vi "App - analyze RUS V6.vi"() -> ()   [LabVIEW 2021] (continued)
s since 1904-01-01), "file name str"="D:\\Data\\Ultrasound\\LSCO\\LSCO22__130814c\\5_Cooling_2nd_try\\September_2014\\091714\\63.35500K_500_2500_2.10000V_0.00000T_Sep17-2014__07-09-10_001_091714.bin", "mod time(min)"=58229949.166666664, "file format"=enum."binary", "power(V)"=2.1, "Magn Field(T) "=0.0}, {"temperature"=63.298, "temperature str"="63.29800", "file path"=path "D:/Data/Ultrasound/LSCO/LSCO22__130814c/5_Cooling_2nd_try/September_2014/091714/63.29800K_500_2500_2.10000V_0.00000T_Sep17-2014__07-10-30_001_091714.bin", "last mod"=timestamp(3493797030 s since 1904-01-01), "file name str"="D:\\Data\\Ultrasound\\LSCO\\LSCO22__130814c\\5_Cooling_2nd_try\\September_2014\\091714\\63.29800K_500_2500_2.10000V_0.00000T_Sep17-2014__07-10-30_001_091714.bin", "mod time(min)"=58229950.5, "file format"=enum."binary", "power(V)"=2.1, "Magn Field(T) "=0.0}, {"temperature"=63.239, "temperature str"="63.23900", "file path"=path "D:/Data/Ultrasound/LSCO/LSCO22__130814c/5_Cooling_2nd_try/September_2014/091714/63.23900K_500_2500_2.10000V_0.00000T_Sep17-2014__07-11-49_001_091714.bin", "last mod"=timestamp(3493797109 s since 1904-01-01), "file name str"="D:\\Data\\Ultrasound\\LSCO\\LSCO22__130814c\\5_Cooling_2nd_try\\September_2014\\091714\\63.23900K_500_2500_2.10000V_0.00000T_Sep17-2014__07-11-49_001_091714.bin", "mod time(min)"=58229951.81666667, "file format"=enum."binary", "power(V)"=2.1, "Magn Field(T) "=0.0}, {"temperature"=63.178, "temperature str"="63.17800", "file path"=path "D:/Data/Ultrasound/LSCO/LSCO22__130814c/5_Cooling_2nd_try/September_2014/091714/63.17800K_500_2500_2.10000V_0.00000T_Sep17-2014__07-13-08_001_091714.bin", "last mod"=timestamp(3493797188 s since 1904-01-01), "file name str"="D:\\Data\\Ultrasound\\LSCO\\LSCO22__130814c\\5_Cooling_2nd_try\\September_2014\\091714\\63.17800K_500_2500_2.10000V_0.00000T_Sep17-2014__07-13-08_001_091714.bin", "mod time(min)"=58229953.13333333, "file format"=enum."binary", "power(V)"=2.1, "Magn Field(T) "=0.0}, {"temperature"=63.123, "temperature str"="63.12300", "file path"=path "D:/Data/Ultrasound/LSCO/LSCO22__130814c/5_Cooling_2nd_try/September_2014/091714/63.12300K_500_2500_2.10000V_0.00000T_Sep17-2014__07-14-28_001_091714.bin", "last mod"=timestamp(3493797268 s since 1904-01-01), "file name str"="D:\\Data\\Ultrasound\\LSCO\\LSCO22__130814c\\5_Cooling_2nd_try\\September_2014\\091714\\63.12300K_500_2500_2.10000V_0.00000T_Sep17-2014__07-14-28_001_091714.bin", "mod time(min)"=58229954.46666667, "file format"=enum."binary", "power(V)"=2.1, "Magn Field(T) "=0.0}, {"temperature"=63.063, "temperature str"="63.06300", "file path"=path "D:/Data/Ultrasound/LSCO/LSCO22__130814c/5_Cooling_2nd_try/September_2014/091714/63.06300K_500_2500_2.10000V_0.00000T_Sep17-2014__07-15-47_001_091714.bin", "last mod"=timestamp(3493797347 s since 1904-01-01), "file name str"="D:\\Data\\Ultrasound\\LSCO\\LSCO22__130814c\\5_Cooling_2nd_try\\September_2014\\091714\\63.06300K_500_2500_2.10000V_0.00000T_Sep17-2014__07-15-47_001_091714.bin", "mod time(min)"=58229955.78333333, "file format"=enum."binary", "power(V)"=2.1, "Magn Field(T) "=0.0}, {"temperature"=63.004, "temperature str"="63.00400", "file path"=path "D:/Data/Ultrasound/LSCO/LSCO22__130814c/5_Cooling_2nd_try/September_2014/091714/63.00400K_500_2500_2.10000V_0.00000T_Sep17-2014__07-17-07_001_091714.bin", "last mod"=timestamp(3493797427 s since 1904-01-01), "file name str"="D:\\Data\\Ultrasound\\LSCO\\LSCO22__130814c\\5_Cooling_2nd_try\\September_2014\\091714\\63.00400K_500_2500_2.10000V_0.00000T_Sep17-2014__07-17-07_001_091714.bin", "mod time(min)"=58229957.11666667, "file format"=enum."binary", "power(V)"=2.1, "Magn Field(T) "=0.0}, {"temperature"=62.948, "temperature str"="62.94800", "file path"=path "D:/Data/Ultrasound/LSCO/LSCO22__130814c/5_Cooling_2nd_try/September_2014/091714/62.94800K_500_2500_2.10000V_0.00000T_Sep17-2014__07-18-26_001_091714.bin", "last mod"=timestamp(3493797506 s since 1904-01-01), "file name str"="D:\\Data\\Ultrasound\\LSCO\\LSCO22__130814c\\5_Cooling_2nd_try\\September_2014\\091714\\62.94800K_500_2500_2.10000V_0.00000T_Sep17-2014__07-18-26_001_091714.bin", "mod time(min)"=58229958.43333333, "file format"=enum."binary", "power(V)"=2.1, "Magn Field(T) "=0.0}, {"temperature"=62.886, "temperature str"="62.88600", "file path"=path "D:/Data/Ultrasound/LSCO/LSCO22__130814c/5_Cooling_2nd_try/September_2014/091714/62.88600K_500_2500_2.10000V_0.00000T_Sep17-2014__07-19-45_001_091714.bin", "last mod"=timestamp(3493797585 s since 1904-01-01), "file name str"="D:\\Data\\Ultrasound\\LSCO\\LSCO22__130814c\\5_Cooling_2nd_try\\September_2014\\091714\\62.88600K_500_2500_2.10000V_0.00000T_Sep17-2014__07-19-45_001_091714.bin", "mod time(min)"=58229959.75, "file format"=enum."binary", "power(V)"=2.1, "Magn Field(T) "=0.0}, {"temperature"=62.828, "temperature str"="62.82800", "file path"=path "D:/Data/Ultrasound/LSCO/LSCO22__130814c/5_Cooling_2nd_try/September_2014/091714/62.82800K_500_2500_2.10000V_0.00000T_Sep17-2014__07-21-05_001_091714.bin", "last mod"=timestamp(3493797665 s since 1904-01-01), "file name str"="D:\\Data\\Ultrasound\\LSCO\\LSCO22__130814c\\5_Cooling_2nd_try\\September_2014\\091714\\62.82800K_500_2500_2.10000V_0.00000T_Sep17-2014__07-21-05_001_091714.bin", "mod time(min)"=58229961.083333336, "file format"=enum."binary", "power(V)"=2.1, "Magn Field(T) "=0.0}, {"temperature"=62.769, "temperature str"="62.76900", "file path"=path "D:/Data/Ultrasound/LSCO/LSCO22__130814c/5_Cooling_2nd_try/September_2014/091714/62.76900K_500_2500_2.10000V_0.00000T_Sep17-2014__07-22-24_001_091714.bin", "last mod"=timestamp(3493797744 s since 1904-01-01), "file name str"="D:\\Data\\Ultrasound\\LSCO\\LSCO22__130814c\\5_Cooling_2nd_try\\September_2014\\091714\\62.76900K_500_2500_2.10000V_0.00000T_Sep17-2014__07-22-24_001_091714.bin", "mod time(min)"=58229962.4, "file format"=enum."binary", "power(V)"=2.1, "Magn Field(T) "=0.0}, {"temperature"=62.713, "temperature str"="62.71300", "file path"=path "D:/Data/Ultrasound/LSCO/LSCO22__130814c/5_Cooling_2nd_try/September_2014/091714/62.71300K_500_2500_2.10000V_0.00000T_Sep17-2014__07-23-43_001_091714.bin", "last mod"=timestamp(3493797823 s since 1904-01-01), "file name str"="D:\\Data\\Ultrasound\\LSCO\\LSCO22__130814c\\5_Cooling_2nd_try\\September_2014\\091714\\62.71300K_500_2500_2.10000V_0.00000T_Sep17-2014__07-23-43_001_091714.bin", "mod time(min)"=58229963.71666667, "file format"=enum."binary", "power(V)"=2.1, "Magn Field(T) "=0.0}, {"temperature"=62.654, "temperature str"="62.65400", "file path"=path "D:/Data/Ultrasound/LSCO/LSCO22__130814c/5_Cooling_2nd_try/September_2014/091714/62.65400K_500_2500_2.10000V_0.00000T_Sep17-2014__07-25-03_001_091714.bin", "last mod"=timestamp(3493797903 s since 1904-01-01), "file name str"="D:\\Data\\Ultrasound\\LSCO\\LSCO22__130814c\\5_Cooling_2nd_try\\September_2014\\091714\\62.65400K_500_2500_2.10000V_0.00000T_Sep17-2014__07-25-03_001_091714.bin", "mod time(min)"=58229965.05, "file format"=enum."binary", "power(V)"=2.1, "Magn Field(T) "=0.0}, {"temperature"=62.592, "temperature str"="62.59200", "file path"=path "D:/Data/Ultrasound/LSCO/LSCO22__130814c/5_Cooling_2nd_try/September_2014/091714/62.59200K_500_2500_2.10000V_0.00000T_Sep17-2014__07-26-22_001_091714.bin", "last mod"=timestamp(3493797982 s since 1904-01-01), "file name str"="D:\\Data\\Ultrasound\\LSCO\\LSCO22__130814c\\5_Cooling_2nd_try\\September_2014\\091714\\62.59200K_500_2500_2.10000V_0.00000T_Sep17-2014__07-26-22_001_091714.bin", "mod time(min)"=58229966.36666667, "file format"=enum."binary", "power(V)"=2.1, "Magn Field(T) "=0.0}, {"temperature"=62.537, "temperature str"="62.53700", "file path"=path "D:/Data/Ultrasound/LSCO/LSCO22__130814c/5_Cooling_2nd_try/September_2014/091714/62.53700K_500_2500_2.10000V_0.00000T_Sep17-2014__07-27-42_001_091714.bin", "last mod"=timestamp(3493798062 s since 1904-01-01), "file name str"="D:\\Data\\Ultrasound\\LSCO\\LSCO22__130814c\\5_Cooling_2nd_try\\September_2014\\091714\\62.53700K_500_2500_2.10000V_0.00000T_Sep17-2014__07-27-42_001_091714.bin", "mod time(min)"=58229967.7, "file format"=enum."binary", "power(V)"=2.1, "Magn Field(T) "=0.0}, {"temperature"=62.48, "temperature str"="62.48000", "file path"=path "D:/Data/Ultrasound/LSCO/LSCO22__130814c/5_Cooling_2nd_try/September_2014/091714/62.48000K_500_2500_2.10000V_0.00000T_Sep17-2014__07-29-01_001_091714.bin", "last mod"=timestamp(3493798141 s since 1904-01-01), "file name str"="D:\\Data\\Ultrasound\\LSCO\\LSCO22__130814c\\5_Cooling_2nd_try\\September_2014\\091714\\62.48000K_500_2500_2.10000V_0.00000T_Sep17-2014__07-29-01_001_091714.bin", "mod time(min)"=58229969.016666666, "file format"=enum."binary", "power(V)"=2.1, "Magn Field(T) "=0.0}, {"temperature"=62.42, "temperature str"="62.42000", "file path"=path "D:/Data/Ultrasound/LSCO/LSCO22__130814c/5_Cooling_2nd_try/September_2014/091714/62.42000K_500_2500_2.10000V_0.00000T_Sep17-2014__07-30-20_001_091714.bin", "last mod"=timestamp(3493798220 s since 1904-01-01), "file name str"="D:\\Data\\Ultrasound\\LSCO\\LSCO22__130814c\\5_Cooling_2nd_try\\September_2014\\091714\\62.42000K_500_2500_2.10000V_0.00000T_Sep17-2014__07-30-20_001_091714.bin", "mod time(min)"=58229970.333333336, "file format"=enum."binary", "power(V)"=2.1, "Magn Field(T) "=0.0}, {"temperature"=62.361, "temperature str"="62.36100", "file path"=path "D:/Data/Ultrasound/LSCO/LSCO22__130814c/5_Cooling_2nd_try/September_2014/091714/62.36100K_500_2500_2.10000V_0.00000T_Sep17-2014__07-31-40_001_091714.bin", "last mod"=timestamp(3493798300 s since 1904-01-01), "file name str"="D:\\Data\\Ultrasound\\LSCO\\LSCO22__130814c\\5_Cooling_2nd_try\\September_2014\\091714\\62.36100K_500_2500_2.10000V_0.00000T_Sep17-2014__07-31-40_001_091714.bin", "mod time(min)"=58229971.666666664, "file format"=enum."binary", "power(V)"=2.1, "Magn Field(T) "=0.0}, {"temperature"=62.301, "temperature str"="62.30100", "file path"=path "D:/Data/Ultrasound/LSCO/LSCO22__130814c/5_Cooling_2nd_try/September_2014/091714/62.30100K_500_2500_2.10000V_0.00000T_Sep17-2014__07-32-59_001_091714.bin", "last mod"=timestamp(3493798379 s since 1904-01-01), "file name str"="D:\\Data\\Ultrasound\\LSCO\\LSCO22__130814c\\5_Cooling_2nd_try\\September_2014\\091714\\62.30100K_500_2500_2.10000V_0.00000T_Sep17-2014__07-32-59_001_091714.bin", "mod time(min)"=58229972.983333334, "file format"=enum."binary", "power(V)"=2.1, "Magn Field(T) "=0.0}, {"temperature"=62.245, "temperature str"="62.24500", "file path"=path "D:/Data/Ultrasound/LSCO/LSCO22__130814c/5_Cooling_2nd_try/September_2014/091714/62.24500K_500_2500_2.10000V_0.00000T_Sep17-2014__07-34-19_001_091714.bin", "last mod"=timestamp(3493798459 s since 1904-01-01), "file name str"="D:\\Data\\Ultrasound\\LSCO\\LSCO22__130814c\\5_Cooling_2nd_try\\September_2014\\091714\\62.24500K_500_2500_2.10000V_0.00000T_Sep17-2014__07-34-19_001_091714.bin", "mod time(min)"=58229974.31666667, "file format"=enum."binary", "power(V)"=2.1, "Magn Field(T) "=0.0}, {"temperature"=62.184, "temperature str"="62.18400", "file path"=path "D:/Data/Ultrasound/LSCO/LSCO22__130814c/5_Cooling_2nd_try/September_2014/091714/62.18400K_500_2500_2.10000V_0.00000T_Sep17-2014__07-35-38_001_091714.bin", "last mod"=timestamp(3493798538 s since 1904-01-01), "file name str"="D:\\Data\\Ultrasound\\LSCO\\LSCO22__130814c\\5_Cooling_2nd_try\\September_2014\\091714\\62.18400K_500_2500_2.10000V_0.00000T_Sep17-2014__07-35-38_001_091714.bin", "mod time(min)"=58229975.63333333, "file format"=enum."binary", "power(V)"=2.1, "Magn Field(T) "=0.0}, {"temperature"=62.127, "temperature str"="62.12700", "file path"=path "D:/Data/Ultrasound/LSCO/LSCO22__130814c/5_Cooling_2nd_try/September_2014/091714/62.12700K_500_2500_2.10000V_0.00000T_Sep17-2014__07-36-57_001_091714.bin", "last mod"=timestamp(3493798617 s since 1904-01-01), "file name str"="D:\\Data\\Ultrasound\\LSCO\\LSCO22__130814c\\5_Cooling_2nd_try\\September_2014\\091714\\62.12700K_500_2500_2.10000V_0.00000T_Sep17-2014__07-36-57_001_091714.bin", "mod time(min)"=58229976.95, "file format"=enum."binary", "power(V)"=2.1, "Magn Field(T) "=0.0}, {"temperature"=62.069, "temperature str"="62.06900", "file path"=path "D:/Data/Ultrasound/LSCO/LSCO22__130814c/5_Cooling_2nd_try/September_2014/091714/62.06900K_500_2500_2.10000V_0.00000T_Sep17-2014__07-38-17_001_091714.bin", "last mod"=timestamp(3493798697 s since 1904-01-01), "file name str"="D:\\Data\\Ultrasound\\LSCO\\LSCO22__130814c\\5_Cooling_2nd_try\\September_2014\\091714\\62.06900K_500_2500_2.10000V_0.00000T_Sep17-2014__07-38-17_001_091714.bin", "mod time(min)"=58229978.28333333, "file format"=enum."binary", "power(V)"=2.1, "Magn Field(T) "=0.0}, {"temperature"=62.01, "temperature str"="62.01000", "file path"=path "D:/Data/Ultrasound/LSCO/LSCO22__130814c/5_Cooling_2nd_try/September_2014/091714/62.01000K_500_2500_2.10000V_0.00000T_Sep17-2014__07-39-36_001_091714.bin", "last mod"=timestamp(3493798776 s since 1904-01-01), "file name str"="D:\\Data\\Ultrasound\\LSCO\\LSCO22__130814c\\5_Cooling_2nd_try\\September_2014\\091714\\62.01000K_500_2500_2.10000V_0.00000T_Sep17-2014__07-39-36_001_091714.bin", "mod time(min)"=58229979.6, "file format"=enum."binary", "power(V)"=2.1, "Magn Field(T) "=0.0}, {"temperature"=61.951, "temperature str"="61.95100", "file path"=path "D:/Data/Ultrasound/LSCO/LSCO22__130814c/5_Cooling_2nd_try/September_2014/091714/61.95100K_500_2500_2.10000V_0.00000T_Sep17-2014__07-40-55_001_091714.bin", "last mod"=timestamp(3493798855 s since 1904-01-01), "file name str"="D:\\Data\\Ultrasound\\LSCO\\LSCO22__130814c\\5_Cooling_2nd_try\\September_2014\\091714\\61.95100K_500_2500_2.10000V_0.00000T_Sep17-2014__07-40-55_001_091714.bin", "mod time(min)"=58229980.916666664, "file format"=enum."binary", "power(V)"=2.1, "Magn Field(T) "=0.0}, {"temperature"=61.895, "temperature str"="61.89500", "file path"=path "D:/Data/Ultrasound/LSCO/LSCO22__130814c/5_Cooling_2nd_try/September_2014/091714/61.89500K_500_2500_2.10000V_0.00000T_Sep17-2014__07-42-15_001_091714.bin", "last mod"=timestamp(3493798935 s since 1904-01-01), "file name str"="D:\\Data\\Ultrasound\\LSCO\\LSCO22__130814c\\5_Cooling_2nd_try\\September_2014\\091714\\61.89500K_500_2500_2.10000V_0.00000T_Sep17-2014__07-42-15_001_091714.bin", "mod time(min)"=58229982.25, "file format"=enum."binary", "power(V)"=2.1, "Magn Field(T) "=0.0}, {"temperature"=61.834, "temperature str"="61.83400", "file path"=path "D:/Data/Ultrasound/LSCO/LSCO22__130814c/5_Cooling_2nd_try/September_2014/091714/61.83400K_500_2500_2.10000V_0.00000T_Sep17-2014__07-43-34_001_091714.bin", "last mod"=timestamp(3493799014 s since 1904-01-01), "file name str"="D:\\Data\\Ultrasound\\LSCO\\LSCO22__130814c\\5_Cooling_2nd_try\\September_2014\\091714\\61.83400K_500_2500_2.10000V_0.00000T_Sep17-2014__07-43-34_001_091714.bin", "mod time(min)"=58229983.56666667, "file format"=enum."binary", "power(V)"=2.1, "Magn Field(T) "=0.0}, {"temperature"=61.775, "temperature str"="61.77500", "file path"=path "D:/Data/Ultrasound/LSCO/LSCO22__130814c/5_Cooling_2nd_try/September_2014/091714/61.77500K_500_2500_2.10000V_0.00000T_Sep17-2014__07-44-54_001_091714.bin", "last mod"=timestamp(3493799094 s since 1904-01-01), "file name str"="D:\\Data\\Ultrasound\\LSCO\\LSCO22__130814c\\5_Cooling_2nd_try\\September_2014\\091714\\61.77500K_500_2500_2.10000V_0.00000T_Sep17-2014__07-44-54_001_091714.bin", "mod time(min)"=58229984.9, "file format"=enum."binary", "power(V)"=2.1, "Magn Field(T) "=0.0}, {"temperature"=61.716, "temperature str"="61.71600", "file path"=path "D:/Data/Ultrasound/LSCO/LSCO22__130814c/5_Cooling_2nd_try/September_2014/091714/61.71600K_500_2500_2.10000V_0.00000T_Sep17-2014__07-46-13_001_091714.bin", "last mod"=timestamp(3493799173 s since 1904-01-01), "file name str"="D:\\Data\\Ultrasound\\LSCO\\LSCO22__130814c\\5_Cooling_2nd_try\\September_2014\\091714\\61.71600K_500_2500_2.10000V_0.00000T_Sep17-2014__07-46-13_001_091714.bin", "mod time(min)"=58229986.21666667, "file format"=enum."binary", "power(V)"=2.1, "Magn Field(T) "=0.0}, {"temperature"=61.656, "temperature str"="61.65600", "file path"=path "D:/Data/Ultrasound/LSCO/LSCO22__130814c/5_Cooling_2nd_try/September_2014/091714/61.65600K_500_2500_2.10000V_0.00000T_Sep17-2014__07-47-32_001_091714.bin", "last mod"=timestamp(3493799252 s since 1904-01-01), "file name str"="D:\\Data\\Ultrasound\\LSCO\\LSCO22__130814c\\5_Cooling_2nd_try\\September_2014\\091714\\61.65600K_500_2500_2.10000V_0.00000T_Sep17-2014__07-47-32_001_091714.bin", "mod time(min)"=58229987.53333333, "file format"=enum."binary", "power(V)"=2.1, "Magn Field(T) "=0.0}, {"temperature"=61.601, "temperature str"="61.60100", "file path"=path "D:/Data/Ultrasound/LSCO/LSCO22__130814c/5_Cooling_2nd_try/September_2014/091714/61.60100K_500_2500_2.10000V_0.00000T_Sep17-2014__07-48-52_001_091714.bin", "last mod"=timestamp(3493799332 s since 1904-01-01), "file name str"="D:\\Data\\Ultrasound\\LSCO\\LSCO22__130814c\\5_Cooling_2nd_try\\September_2014\\091714\\61.60100K_500_2500_2.10000V_0.00000T_Sep17-2014__07-48-52_001_091714.bin", "mod time(min)"=58229988.86666667, "file format"=enum."binary", "power(V)"=2.1, "Magn Field(T) "=0.0}, {"temperature"=61.541, "temperature str"="61.54100", "file path"=path "D:/Data/Ultrasound/LSCO/LSCO22__130814c/5_Cooling_2nd_try/September_2014/091714/61.54100K_500_2500_2.10000V_0.00000T_Sep17-2014__07-50-11_001_091714.bin", "last mod"=timestamp(3493799411 s since 1904-01-01), "file name str"="D:\\Data\\Ultrasound\\LSCO\\LSCO22__130814c\\5_Cooling_2nd_try\\September_2014\\091714\\61.54100K_500_2500_2.10000V_0.00000T_Sep17-2014__07-50-11_001_091714.bin", "mod time(min)"=58229990.18333333, "file format"=enum."binary", "power(V)"=2.1, "Magn Field(T) "=0.0}, {"temperature"=61.482, "temperature str"="61.48200", "file path"=path "D:/Data/Ultrasound/LSCO/LSCO22__130814c/5_Cooling_2nd_try/September_2014/091714/61.48200K_500_2500_2.10000V_0.00000T_Sep17-2014__07-51-31_001_091714.bin", "last mod"=timestamp(3493799491 s since 1904-01-01), "file name str"="D:\\Data\\Ultrasound\\LSCO\\LSCO22__130814c\\5_Cooling_2nd_try\\September_2014\\091714\\61.48200K_500_2500_2.10000V_0.00000T_Sep17-2014__07-51-31_001_091714.bin", "mod time(min)"=58229991.516666666, "file format"=enum."binary", "power(V)"=2.1, "Magn Field(T) "=0.0}, {"temperature"=61.424, "temperature str"="61.42400", "file path"=path "D:/Data/Ultrasound/LSCO/LSCO22__130814c/5_Cooling_2nd_try/September_2014/091714/61.42400K_500_2500_2.10000V_0.00000T_Sep17-2014__07-52-50_001_091714.bin", "last mod"=timestamp(3493799570 s since 1904-01-01), "file name str"="D:\\Data\\Ultrasound\\LSCO\\LSCO22__130814c\\5_Cooling_2nd_try\\September_2014\\091714\\61.42400K_500_2500_2.10000V_0.00000T_Sep17-2014__07-52-50_001_091714.bin", "mod time(min)"=58229992.833333336, "file format"=enum."binary", "power(V)"=2.1, "Magn Field(T) "=0.0}, {"temperature"=61.367, "temperature str"="61.36700", "file path"=path "D:/Data/Ultrasound/LSCO/LSCO22__130814c/5_Cooling_2nd_try/September_2014/091714/61.36700K_500_2500_2.10000V_0.00000T_Sep17-2014__07-54-09_001_091714.bin", "last mod"=timestamp(3493799649 s since 1904-01-01), "file name str"="D:\\Data\\Ultrasound\\LSCO\\LSCO22__130814c\\5_Cooling_2nd_try\\September_2014\\091714\\61.36700K_500_2500_2.10000V_0.00000T_Sep17-2014__07-54-09_001_091714.bin", "mod time(min)"=58229994.15, "file format"=enum."binary", "power(V)"=2.1, "Magn Field(T) "=0.0}, {"temperature"=61.307, "temperature str"="61.30700", "file path"=path "D:/Data/Ultrasound/LSCO/LSCO22__130814c/5_Cooling_2nd_try/September_2014/091714/61.30700K_500_2500_2.10000V_0.00000T_Sep17-2014__07-55-29_001_091714.bin", "last mod"=timestamp(3493799729 s since 1904-01-01), "file name str"="D:\\Data\\Ultrasound\\LSCO\\LSCO22__130814c\\5_Cooling_2nd_try\\September_2014\\091714\\61.30700K_500_2500_2.10000V_0.00000T_Sep17-2014__07-55-29_001_091714.bin", "mod time(min)"=58229995.483333334, "file format"=enum."binary", "power(V)"=2.1, "Magn Field(T) "=0.0}, {"temperature"=61.247, "temperature str"="61.24700", "file path"=path "D:/Data/Ultrasound/LSCO/LSCO22__130814c/5_Cooling_2nd_try/September_2014/091714/61.24700K_500_2500_2.10000V_0.00000T_Sep17-2014__07-56-48_001_091714.bin", "last mod"=timestamp(3493799808 s since 1904-01-01), "file name str"="D:\\Data\\Ultrasound\\LSCO\\LSCO22__130814c\\5_Cooling_2nd_try\\September_2014\\091714\\61.24700K_500_2500_2.10000V_0.00000T_Sep17-2014__07-56-48_001_091714.bin", "mod time(min)"=58229996.8, "file format"=enum."binary", "power(V)"=2.1, "Magn Field(T) "=0.0}, {"temperature"=61.191, "temperature str"="61.19100", "file path"=path "D:/Data/Ultrasound/LSCO/LSCO22__130814c/5_Cooling_2nd_try/September_2014/091714/61.19100K_500_2500_2.10000V_0.00000T_Sep17-2014__07-58-07_001_091714.bin", "last mod"=timestamp(3493799887 s since 1904-01-01), "file name str"="D:\\Data\\Ultrasound\\LSCO\\LSCO22__130814c\\5_Cooling_2nd_try\\September_2014\\091714\\61.19100K_500_2500_2.10000V_0.00000T_Sep17-2014__07-58-07_001_091714.bin", "mod time(min)"=58229998.11666667, "file format"=enum."binary", "power(V)"=2.1, "Magn Field(T) "=0.0}, {"temperature"=61.13, "temperature str"="61.13000", "file path"=path "D:/Data/Ultrasound/LSCO/LSCO22__130814c/5_Cooling_2nd_try/September_2014/091714/61.13000K_500_2500_2.10000V_0.00000T_Sep17-2014__07-59-27_001_091714.bin", "last mod"=timestamp(3493799967 s since 1904-01-01), "file name str"="D:\\Data\\Ultrasound\\LSCO\\LSCO22__130814c\\5_Cooling_2nd_try\\September_2014\\091714\\61.13000K_500_2500_2.10000V_0.00000T_Sep17-2014__07-59-27_001_091714.bin", "mod time(min)"=58229999.45, "file format"=enum."binary", "power(V)"=2.1, "Magn Field(T) "=0.0}, {"temperature"=61.073, "temperature str"="61.07300", "file path"=path "D:/Data/Ultrasound/LSCO/LSCO22__130814c/5_Cooling_2nd_try/September_2014/091714/61.07300K_500_2500_2.10000V_0.00000T_Sep17-2014__08-00-46_001_091714.bin", "last mod"=timestamp(3493800046 s since 1904-01-01), "file name str"="D:\\Data\\Ultrasound\\LSCO\\LSCO22__130814c\\5_Cooling_2nd_try\\September_2014\\091714\\61.07300K_500_2500_2.10000V_0.00000T_Sep17-2014__08-00-46_001_091714.bin", "mod time(min)"=58230000.766666666, "file format"=enum."binary", "power(V)"=2.1, "Magn Field(T) "=0.0}, {"temperature"=61.013, "temperature str"="61.01300", "file path"=path "D:/Data/Ultrasound/LSCO/LSCO22__130814c/5_Cooling_2nd_try/September_2014/091714/61.01300K_500_2500_2.10000V_0.00000T_Sep17-2014__08-02-06_001_091714.bin", "last mod"=timestamp(3493800126 s since 1904-01-01), "file name str"="D:\\Data\\Ultrasound\\LSCO\\LSCO22__130814c\\5_Cooling_2nd_try\\September_2014\\091714\\61.01300K_500_2500_2.10000V_0.00000T_Sep17-2014__08-02-06_001_091714.bin", "mod time(min)"=58230002.1, "file format"=enum."binary", "power(V)"=2.1, "Magn Field(T) "=0.0}, {"temperature"=60.953, "temperature str"="60.95300", "file path"=path "D:/Data/Ultrasound/LSCO/LSCO22__130814c/5_Cooling_2nd_try/September_2014/091714/60.95300K_500_2500_2.10000V_0.00000T_Sep17-2014__08-03-25_001_091714.bin", "last mod"=timestamp(3493800205 s since 1904-01-01), "file name str"="D:\\Data\\Ultrasound\\LSCO\\LSCO22__130814c\\5_Cooling_2nd_try\\September_2014\\091714\\60.95300K_500_2500_2.10000V_0.00000T_Sep17-2014__08-03-25_001_091714.bin", "mod time(min)"=58230003.416666664, "file format"=enum."binary", "power(V)"=2.1, "Magn Field(T) "=0.0}, {"temperature"=60.896, "temperature str"="60.89600", "file path"=path "D:/Data/Ultrasound/LSCO/LSCO22__130814c/5_Cooling_2nd_try/September_2014/091714/60.89600K_500_2500_2.10000V_0.00000T_Sep17-2014__08-04-44_001_091714.bin", "last mod"=timestamp(3493800284 s since 1904-01-01), "file name str"="D:\\Data\\Ultrasound\\LSCO\\LSCO22__130814c\\5_Cooling_2nd_try\\September_2014\\091714\\60.89600K_500_2500_2.10000V_0.00000T_Sep17-2014__08-04-44_001_091714.bin", "mod time(min)"=58230004.733333334, "file format"=enum."binary", "power(V)"=2.1, "Magn Field(T) "=0.0}, {"temperature"=60.837, "temperature str"="60.83700", "file path"=path "D:/Data/Ultrasound/LSCO/LSCO22__130814c/5_Cooling_2nd_try/September_2014/091714/60.83700K_500_2500_2.10000V_0.00000T_Sep17-2014__08-06-04_001_091714.bin", "last mod"=timestamp(3493800364 s since 1904-01-01), "file name str"="D:\\Data\\Ultrasound\\LSCO\\LSCO22__130814c\\5_Cooling_2nd_try\\September_2014\\091714\\60.83700K_500_2500_2.10000V_0.00000T_Sep17-2014__08-06-04_001_091714.bin", "mod time(min)"=58230006.06666667, "file format"=enum."binary", "power(V)"=2.1, "Magn Field(T) "=0.0}, {"temperature"=60.781, "temperature str"="60.78100", "file path"=path "D:/Data/Ultrasound/LSCO/LSCO22__130814c/5_Cooling_2nd_try/September_2014/091714/60.78100K_500_2500_2.10000V_0.00000T_Sep17-2014__08-07-23_001_091714.bin", "last mod"=timestamp(3493800443 s since 1904-01-01), "file name str"="D:\\Data\\Ultrasound\\LSCO\\LSCO22__130814c\\5_Cooling_2nd_try\\September_2014\\091714\\60.78100K_500_2500_2.10000V_0.00000T_Sep17-2014__08-07-23_001_091714.bin", "mod time(min)"=58230007.38333333, "file format"=enum."binary", "power(V)"=2.1, "Magn Field(T) "=0.0}, {"temperature"=60.72, "temperature str"="60.72000", "file path"=path "D:/Data/Ultrasound/LSCO/LSCO22__130814c/5_Cooling_2nd_try/September_2014/091714/60.72000K_500_2500_2.10000V_0.00000T_Sep17-2014__08-08-42_001_091714.bin", "last mod"=timestamp(3493800522 s since 1904-01-01), "file name str"="D:\\Data\\Ultrasound\\LSCO\\LSCO22__130814c\\5_Cooling_2nd_try\\September_2014\\091714\\60.72000K_500_2500_2.10000V_0.00000T_Sep17-2014__08-08-42_001_091714.bin", "mod time(min)"=58230008.7, "file format"=enum."binary", "power(V)"=2.1, "Magn Field(T) "=0.0}, {"temperature"=60.659, "temperature str"="60.65900", "file path"=path "D:/Data/Ultrasound/LSCO/LSCO22__130814c/5_Cooling_2nd_try/September_2014/091714/60.65900K_500_2500_2.10000V_0.00000T_Sep17-2014__08-10-02_001_091714.bin", "last mod"=timestamp(3493800602 s since 1904-01-01), "file name str"="D:\\Data\\Ultrasound\\LSCO\\LSCO22__130814c\\5_Cooling_2nd_try\\September_2014\\091714\\60.65900K_500_2500_2.10000V_0.00000T_Sep17-2014__08-10-02_001_091714.bin", "mod time(min)"=58230010.03333333, "file format"=enum."binary", "power(V)"=2.1, "Magn Field(T) "=0.0}, {"temperature"=60.601, "temperature str"="60.60100", "file path"=path "D:/Data/Ultrasound/LSCO/LSCO22__130814c/5_Cooling_2nd_try/September_2014/091714/60.60100K_500_2500_2.10000V_0.00000T_Sep17-2014__08-11-21_001_091714.bin", "last mod"=timestamp(3493800681 s since 1904-01-01), "file name str"="D:\\Data\\Ultrasound\\LSCO\\LSCO22__130814c\\5_Cooling_2nd_try\\September_2014\\091714\\60.60100K_500_2500_2.10000V_0.00000T_Sep17-2014__08-11-21_001_091714.bin", "mod time(min)"=58230011.35, "file format"=enum."binary", "power(V)"=2.1, "Magn Field(T) "=0.0}, {"temperature"=60.545, "temperature str"="60.54500", "file path"=path "D:/Data/Ultrasound/LSCO/LSCO22__130814c/5_Cooling_2nd_try/September_2014/091714/60.54500K_500_2500_2.10000V_0.00000T_Sep17-2014__08-12-41_001_091714.bin", "last mod"=timestamp(3493800761 s since 1904-01-01), "file name str"="D:\\Data\\Ultrasound\\LSCO\\LSCO22__130814c\\5_Cooling_2nd_try\\September_2014\\091714\\60.54500K_500_2500_2.10000V_0.00000T_Sep17-2014__08-12-41_001_091714.bin", "mod time(min)"=58230012.68333333, "file format"=enum."binary", "power(V)"=2.1, "Magn Field(T) "=0.0}, {"temperature"=60.486, "temperature str"="60.48600", "file path"=path "D:/Data/Ultrasound/LSCO/LSCO22__130814c/5_Cooling_2nd_try/September_2014/091714/60.48600K_500_2500_2.10000V_0.00000T_Sep17-2014__08-14-00_001_091714.bin", "last mod"=timestamp(3493800840 s since 1904-01-01), "file name str"="D:\\Data\\Ultrasound\\LSCO\\LSCO22__130814c\\5_Cooling_2nd_try\\September_2014\\091714\\60.48600K_500_2500_2.10000V_0.00000T_Sep17-2014__08-14-00_001_091714.bin", "mod time(min)"=58230014.0, "file format"=enum."binary", "power(V)"=2.1, "Magn Field(T) "=0.0}, {"temperature"=60.426, "temperature str"="60.42600", "file path"=path "D:/Data/Ultrasound/LSCO/LSCO22__130814c/5_Cooling_2nd_try/September_2014/091714/60.42600K_500_2500_2.10000V_0.00000T_Sep17-2014__08-15-19_001_091714.bin", "last mod"=timestamp(3493800919 s since 1904-01-01), "file name str"="D:\\Data\\Ultrasound\\LSCO\\LSCO22__130814c\\5_Cooling_2nd_try\\September_2014\\091714\\60.42600K_500_2500_2.10000V_0.00000T_Sep17-2014__08-15-19_001_091714.bin", "mod time(min)"=58230015.31666667, "file format"=enum."binary", "power(V)"=2.1, "Magn Field(T) "=0.0}, {"temperature"=60.367, "temperature str"="60.36700", "file path"=path "D:/Data/Ultrasound/LSCO/LSCO22__130814c/5_Cooling_2nd_try/September_2014/091714/60.36700K_500_2500_2.10000V_0.00000T_Sep17-2014__08-16-39_001_091714.bin", "last mod"=timestamp(3493800999 s since 1904-01-01), "file name str"="D:\\Data\\Ultrasound\\LSCO\\LSCO22__130814c\\5_Cooling_2nd_try\\September_2014\\091714\\60.36700K_500_2500_2.10000V_0.00000T_Sep17-2014__08-16-39_001_091714.bin", "mod time(min)"=58230016.65, "file format"=enum."binary", "power(V)"=2.1, "Magn Field(T) "=0.0}, {"temperature"=60.308, "temperature str"="60.30800", "file path"=path "D:/Data/Ultrasound/LSCO/LSCO22__130814c/5_Cooling_2nd_try/September_2014/091714/60.30800K_500_2500_2.10000V_0.00000T_Sep17-2014__08-17-58_001_091714.bin", "last mod"=timestamp(3493801078 s since 1904-01-01), "file name str"="D:\\Data\\Ultrasound\\LSCO\\LSCO22__130814c\\5_Cooling_2nd_try\\September_2014\\091714\\60.30800K_500_2500_2.10000V_0.00000T_Sep17-2014__08-17-58_001_091714.bin", "mod time(min)"=58230017.96666667, "file format"=enum."binary", "power(V)"=2.1, "Magn Field(T) "=0.0}, {"temperature"=60.248, "temperature str"="60.24800", "file path"=path "D:/Data/Ultrasound/LSCO/LSCO22__130814c/5_Cooling_2nd_try/September_2014/091714/60.24800K_500_2500_2.10000V_0.00000T_Sep17-2014__08-19-18_001_091714.bin", "last mod"=timestamp(3493801158 s since 1904-01-01), "file name str"="D:\\Data\\Ultrasound\\LSCO\\LSCO22__130814c\\5_Cooling_2nd_try\\September_2014\\091714\\60.24800K_500_2500_2.10000V_0.00000T_Sep17-2014__08-19-18_001_091714.bin", "mod time(min)"=58230019.3, "file format"=enum."binary", "power(V)"=2.1, "Magn Field(T) "=0.0}, {"temperature"=60.19, "temperature str"="60.19000", "file path"=path "D:/Data/Ultrasound/LSCO/LSCO22__130814c/5_Cooling_2nd_try/September_2014/091714/60.19000K_500_2500_2.10000V_0.00000T_Sep17-2014__08-20-37_001_091714.bin", "last mod"=timestamp(3493801237 s since 1904-01-01), "file name str"="D:\\Data\\Ultrasound\\LSCO\\LSCO22__130814c\\5_Cooling_2nd_try\\September_2014\\091714\\60.19000K_500_2500_2.10000V_0.00000T_Sep17-2014__08-20-37_001_091714.bin", "mod time(min)"=58230020.61666667, "file format"=enum."binary", "power(V)"=2.1, "Magn Field(T) "=0.0}, {"temperature"=60.133, "temperature str"="60.13300", "file path"=path "D:/Data/Ultrasound/LSCO/LSCO22__130814c/5_Cooling_2nd_try/September_2014/091714/60.13300K_500_2500_2.10000V_0.00000T_Sep17-2014__08-21-56_001_091714.bin", "last mod"=timestamp(3493801316 s since 1904-01-01), "file name str"="D:\\Data\\Ultrasound\\LSCO\\LSCO22__130814c\\5_Cooling_2nd_try\\September_2014\\091714\\60.13300K_500_2500_2.10000V_0.00000T_Sep17-2014__08-21-56_001_091714.bin", "mod time(min)"=58230021.93333333, "file format"=enum."binary", "power(V)"=2.1, "Magn Field(T) "=0.0}, {"temperature"=60.073, "temperature str"="60.07300", "file path"=path "D:/Data/Ultrasound/LSCO/LSCO22__130814c/5_Cooling_2nd_try/September_2014/091714/60.07300K_500_2500_2.10000V_0.00000T_Sep17-2014__08-23-16_001_091714.bin", "last mod"=timestamp(3493801396 s since 1904-01-01), "file name str"="D:\\Data\\Ultrasound\\LSCO\\LSCO22__130814c\\5_Cooling_2nd_try\\September_2014\\091714\\60.07300K_500_2500_2.10000V_0.00000T_Sep17-2014__08-23-16_001_091714.bin", "mod time(min)"=58230023.266666666, "file format"=enum."binary", "power(V)"=2.1, "Magn Field(T) "=0.0}, {"temperature"=60.013, "temperature str"="60.01300", "file path"=path "D:/Data/Ultrasound/LSCO/LSCO22__130814c/5_Cooling_2nd_try/September_2014/091714/60.01300K_500_2500_2.10000V_0.00000T_Sep17-2014__08-24-35_001_091714.bin", "last mod"=timestamp(3493801475 s since 1904-01-01), "file name str"="D:\\Data\\Ultrasound\\LSCO\\LSCO22__130814c\\5_Cooling_2nd_try\\September_2014\\091714\\60.01300K_500_2500_2.10000V_0.00000T_Sep17-2014__08-24-35_001_091714.bin", "mod time(min)"=58230024.583333336, "file format"=enum."binary", "power(V)"=2.1, "Magn Field(T) "=0.0}, {"temperature"=59.955, "temperature str"="59.95500", "file path"=path "D:/Data/Ultrasound/LSCO/LSCO22__130814c/5_Cooling_2nd_try/September_2014/091714/59.95500K_500_2500_2.10000V_0.00000T_Sep17-2014__08-25-54_001_091714.bin", "last mod"=timestamp(3493801554 s since 1904-01-01), "file name str"="D:\\Data\\Ultrasound\\LSCO\\LSCO22__130814c\\5_Cooling_2nd_try\\September_2014\\091714\\59.95500K_500_2500_2.10000V_0.00000T_Sep17-2014__08-25-54_001_091714.bin", "mod time(min)"=58230025.9, "file format"=enum."binary", "power(V)"=2.1, "Magn Field(T) "=0.0}, {"temperature"=59.894, "temperature str"="59.89400", "file path"=path "D:/Data/Ultrasound/LSCO/LSCO22__130814c/5_Cooling_2nd_try/September_2014/091714/59.89400K_500_2500_2.10000V_0.00000T_Sep17-2014__08-27-14_001_091714.bin", "last mod"=timestamp(3493801634 s since 1904-01-01), "file name str"="D:\\Data\\Ultrasound\\LSCO\\LSCO22__130814c\\5_Cooling_2nd_try\\September_2014\\091714\\59.89400K_500_2500_2.10000V_0.00000T_Sep17-2014__08-27-14_001_091714.bin", "mod time(min)"=58230027.233333334, "file format"=enum."binary", "power(V)"=2.1, "Magn Field(T) "=0.0}, {"temperature"=59.839, "temperature str"="59.83900", "file path"=path "D:/Data/Ultrasound/LSCO/LSCO22__130814c/5_Cooling_2nd_try/September_2014/091714/59.83900K_500_2500_2.10000V_0.00000T_Sep17-2014__08-28-33_001_091714.bin", "last mod"=timestamp(3493801713 s since 1904-01-01), "file name str"="D:\\Data\\Ultrasound\\LSCO\\LSCO22__130814c\\5_Cooling_2nd_try\\September_2014\\091714\\59.83900K_500_2500_2.10000V_0.00000T_Sep17-2014__08-28-33_001_091714.bin", "mod time(min)"=58230028.55, "file format"=enum."binary", "power(V)"=2.1, "Magn Field(T) "=0.0}, {"temperature"=59.776, "temperature str"="59.77600", "file path"=path "D:/Data/Ultrasound/LSCO/LSCO22__130814c/5_Cooling_2nd_try/September_2014/091714/59.77600K_500_2500_2.10000V_0.00000T_Sep17-2014__08-29-53_001_091714.bin", "last mod"=timestamp(3493801793 s since 1904-01-01), "file name str"="D:\\Data\\Ultrasound\\LSCO\\LSCO22__130814c\\5_Cooling_2nd_try\\September_2014\\091714\\59.77600K_500_2500_2.10000V_0.00000T_Sep17-2014__08-29-53_001_091714.bin", "mod time(min)"=58230029.88333333, "file format"=enum."binary", "power(V)"=2.1, "Magn Field(T) "=0.0}, {"temperature"=59.72, "temperature str"="59.72000", "file path"=path "D:/Data/Ultrasound/LSCO/LSCO22__130814c/5_Cooling_2nd_try/September_2014/091714/59.72000K_500_2500_2.10000V_0.00000T_Sep17-2014__08-31-12_001_091714.bin", "last mod"=timestamp(3493801872 s since 1904-01-01), "file name str"="D:\\Data\\Ultrasound\\LSCO\\LSCO22__130814c\\5_Cooling_2nd_try\\September_2014\\091714\\59.72000K_500_2500_2.10000V_0.00000T_Sep17-2014__08-31-12_001_091714.bin", "mod time(min)"=58230031.2, "file format"=enum."binary", "power(V)"=2.1, "Magn Field(T) "=0.0}, {"temperature"=59.661, "temperature str"="59.66100", "file path"=path "D:/Data/Ultrasound/LSCO/LSCO22__130814c/5_Cooling_2nd_try/September_2014/091714/59.66100K_500_2500_2.10000V_0.00000T_Sep17-2014__08-32-31_001_091714.bin", "last mod"=timestamp(3493801951 s since 1904-01-01), "file name str"="D:\\Data\\Ultrasound\\LSCO\\LSCO22__130814c\\5_Cooling_2nd_try\\September_2014\\091714\\59.66100K_500_2500_2.10000V_0.00000T_Sep17-2014__08-32-31_001_091714.bin", "mod time(min)"=58230032.516666666, "file format"=enum."binary", "power(V)"=2.1, "Magn Field(T) "=0.0}, {"temperature"=59.598, "temperature str"="59.59800", "file path"=path "D:/Data/Ultrasound/LSCO/LSCO22__130814c/5_Cooling_2nd_try/September_2014/091714/59.59800K_500_2500_2.10000V_0.00000T_Sep17-2014__08-33-51_001_091714.bin", "last mod"=timestamp(3493802031 s since 1904-01-01), "file name str"="D:\\Data\\Ultrasound\\LSCO\\LSCO22__130814c\\5_Cooling_2nd_try\\September_2014\\091714\\59.59800K_500_2500_2.10000V_0.00000T_Sep17-2014__08-33-51_001_091714.bin", "mod time(min)"=58230033.85, "file format"=enum."binary", "power(V)"=2.1, "Magn Field(T) "=0.0}, {"temperature"=59.54, "temperature str"="59.54000", "file path"=path "D:/Data/Ultrasound/LSCO/LSCO22__130814c/5_Cooling_2nd_try/September_2014/091714/59.54000K_500_2500_2.10000V_0.00000T_Sep17-2014__08-35-10_001_091714.bin", "last mod"=timestamp(3493802110 s since 1904-01-01), "file name str"="D:\\Data\\Ultrasound\\LSCO\\LSCO22__130814c\\5_Cooling_2nd_try\\September_2014\\091714\\59.54000K_500_2500_2.10000V_0.00000T_Sep17-2014__08-35-10_001_091714.bin", "mod time(min)"=58230035.166666664, "file format"=enum."binary", "power(V)"=2.1, "Magn Field(T) "=0.0}, {"temperature"=59.481, "temperature str"="59.48100", "file path"=path "D:/Data/Ultrasound/LSCO/LSCO22__130814c/5_Cooling_2nd_try/September_2014/091714/59.48100K_500_2500_2.10000V_0.00000T_Sep17-2014__08-36-30_001_091714.bin", "last mod"=timestamp(3493802190 s since 1904-01-01), "file name str"="D:\\Data\\Ultrasound\\LSCO\\LSCO22__130814c\\5_Cooling_2nd_try\\September_2014\\091714\\59.48100K_500_2500_2.10000V_0.00000T_Sep17-2014__08-36-30_001_091714.bin", "mod time(min)"=58230036.5, "file format"=enum."binary", "power(V)"=2.1, "Magn Field(T) "=0.0}, {"temperature"=59.422, "temperature str"="59.42200", "file path"=path "D:/Data/Ultrasound/LSCO/LSCO22__130814c/5_Cooling_2nd_try/September_2014/091714/59.42200K_500_2500_2.10000V_0.00000T_Sep17-2014__08-37-49_001_091714.bin", "last mod"=timestamp(3493802269 s since 1904-01-01), "file name str"="D:\\Data\\Ultrasound\\LSCO\\LSCO22__130814c\\5_Cooling_2nd_try\\September_2014\\091714\\59.42200K_500_2500_2.10000V_0.00000T_Sep17-2014__08-37-49_001_091714.bin", "mod time(min)"=58230037.81666667, "file format"=enum."binary", "power(V)"=2.1, "Magn Field(T) "=0.0}, {"temperature"=59.365, "temperature str"="59.36500", "file path"=path "D:/Data/Ultrasound/LSCO/LSCO22__130814c/5_Cooling_2nd_try/September_2014/091714/59.36500K_500_2500_2.10000V_0.00000T_Sep17-2014__08-39-08_001_091714.bin", "last mod"=timestamp(3493802348 s since 1904-01-01), "file name str"="D:\\Data\\Ultrasound\\LSCO\\LSCO22__130814c\\5_Cooling_2nd_try\\September_2014\\091714\\59.36500K_500_2500_2.10000V_0.00000T_Sep17-2014__08-39-08_001_091714.bin", "mod time(min)"=58230039.13333333, "file format"=enum."binary", "power(V)"=2.1, "Magn Field(T) "=0.0}, {"temperature"=59.302, "temperature str"="59.30200", "file path"=path "D:/Data/Ultrasound/LSCO/LSCO22__130814c/5_Cooling_2nd_try/September_2014/091714/59.30200K_500_2500_2.10000V_0.00000T_Sep17-2014__08-40-28_001_091714.bin", "last mod"=timestamp(3493802428 s since 1904-01-01), "file name str"="D:\\Data\\Ultrasound\\LSCO\\LSCO22__130814c\\5_Cooling_2nd_try\\September_2014\\091714\\59.30200K_500_2500_2.10000V_0.00000T_Sep17-2014__08-40-28_001_091714.bin", "mod time(min)"=58230040.46666667, "file format"=enum."binary", "power(V)"=2.1, "Magn Field(T) "=0.0}, {"temperature"=59.243, "temperature str"="59.24300", "file path"=path "D:/Data/Ultrasound/LSCO/LSCO22__130814c/5_Cooling_2nd_try/September_2014/091714/59.24300K_500_2500_2.10000V_0.00000T_Sep17-2014__08-41-47_001_091714.bin", "last mod"=timestamp(3493802507 s since 1904-01-01), "file name str"="D:\\Data\\Ultrasound\\LSCO\\LSCO22__130814c\\5_Cooling_2nd_try\\September_2014\\091714\\59.24300K_500_2500_2.10000V_0.00000T_Sep17-2014__08-41-47_001_091714.bin", "mod time(min)"=58230041.78333333, "file format"=enum."binary", "power(V)"=2.1, "Magn Field(T) "=0.0}, {"temperature"=59.186, "temperature str"="59.18600", "file path"=path "D:/Data/Ultrasound/LSCO/LSCO22__130814c/5_Cooling_2nd_try/September_2014/091714/59.18600K_500_2500_2.10000V_0.00000T_Sep17-2014__08-43-06_001_091714.bin", "last mod"=timestamp(3493802586 s since 1904-01-01), "file name str"="D:\\Data\\Ultrasound\\LSCO\\LSCO22__130814c\\5_Cooling_2nd_try\\September_2014\\091714\\59.18600K_500_2500_2.10000V_0.00000T_Sep17-2014__08-43-06_001_091714.bin", "mod time(min)"=58230043.1, "file format"=enum."binary", "power(V)"=2.1, "Magn Field(T) "=0.0}, 
